vi "Evaluate Single Solution.vi"(7 "Processing Times (Rows Mach.Cols Jobs)":u16[][](array[numeric]), 9 "Schedule":u16[](array[numeric]), 10 "Number of Jobs":i32, 11 "Number of Machines":i32) -> (3 "Gannt Chart Out":T1[][](array[typedef]))   [LabVIEW 2013, in "GA.lvclass"]
uses:
  GA.lvclass
  Controls/GanntChart_Element.ctl
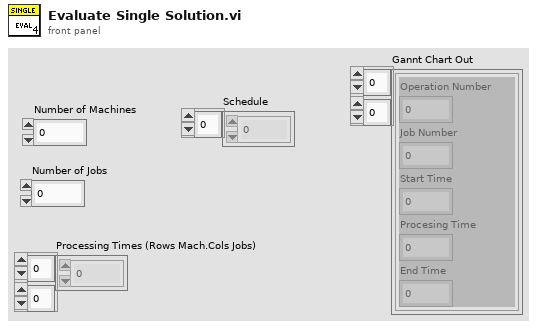
[diagram p1: front panel]
types:
  T1 = typedef "GanntChart_Element.ctl" = cluster{"Operation Number":i32, "Job Number":i32, "Start Time":i32, "Procesing Time":u16, "End Time":i32}
  T2 = typedef "Time_Interval_List_Element.ctl" = cluster{"Start Time":i32, "End Time":i32}
  T3 = typedef "Gap.ctl" = cluster{"Gap Start Time":i32, "Gap End Time":i32, "Gap Index":i32}
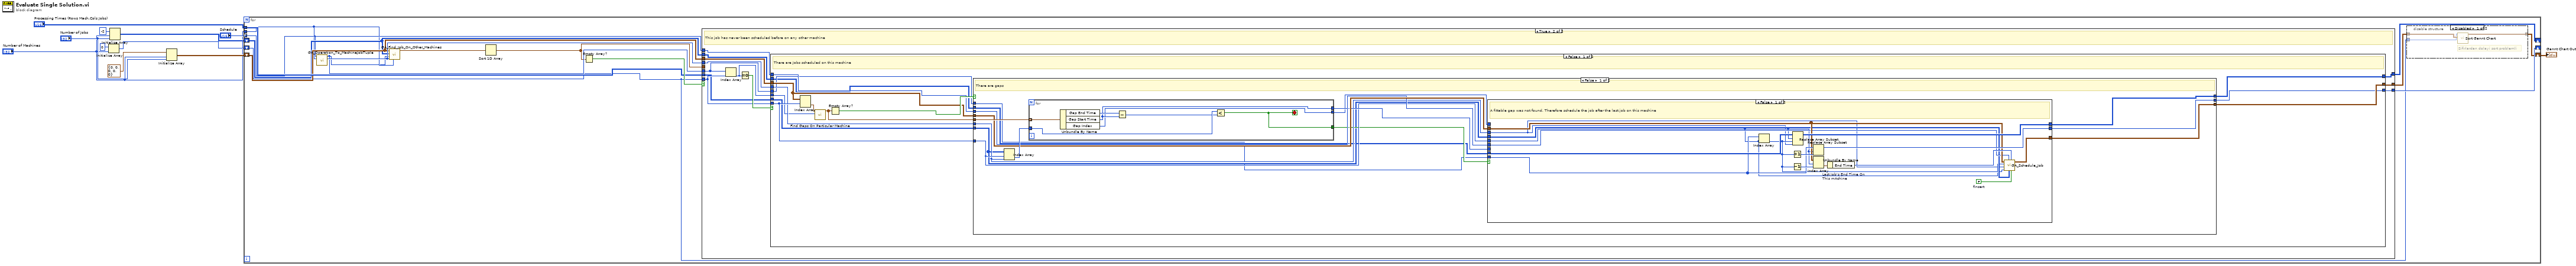
[diagram p0: block diagram]
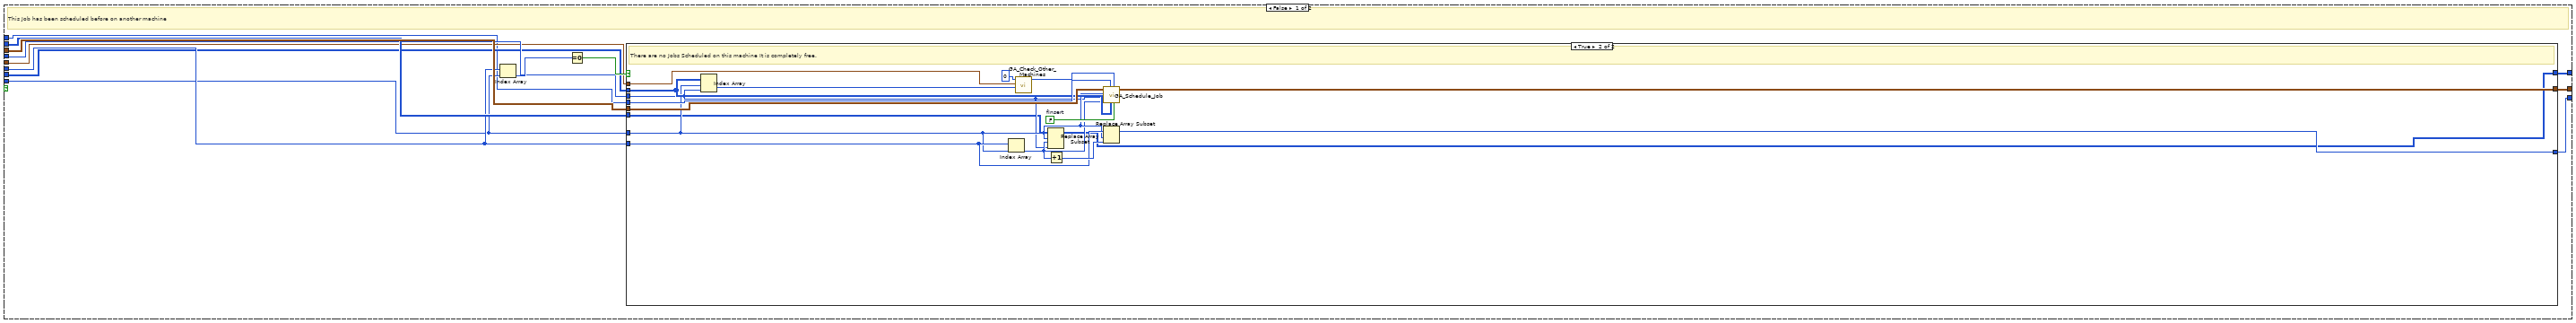
[diagram p3: hidden frame]
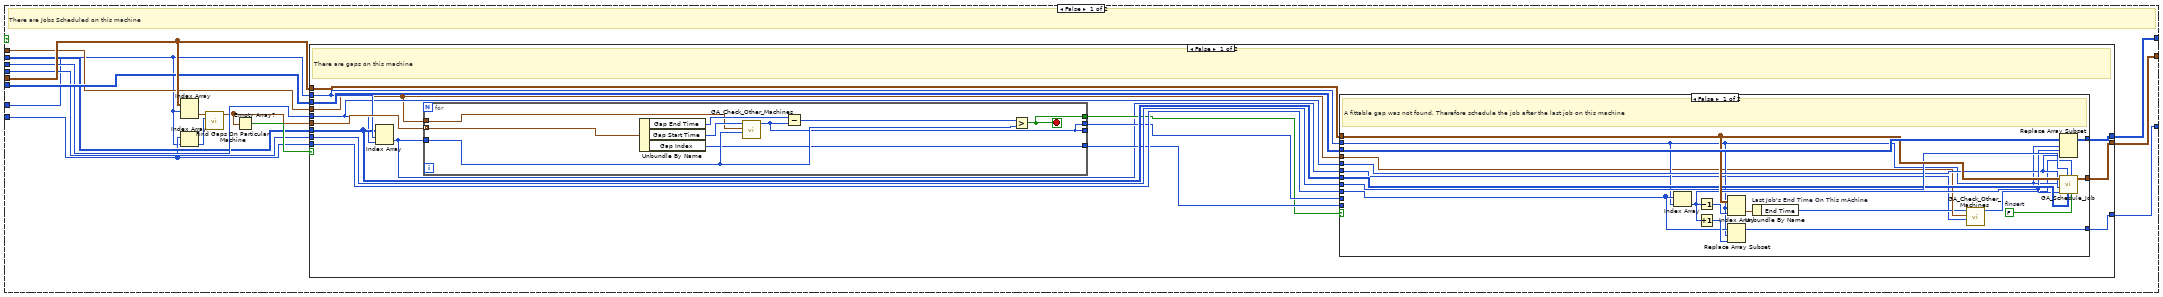
[diagram p4: hidden frame]
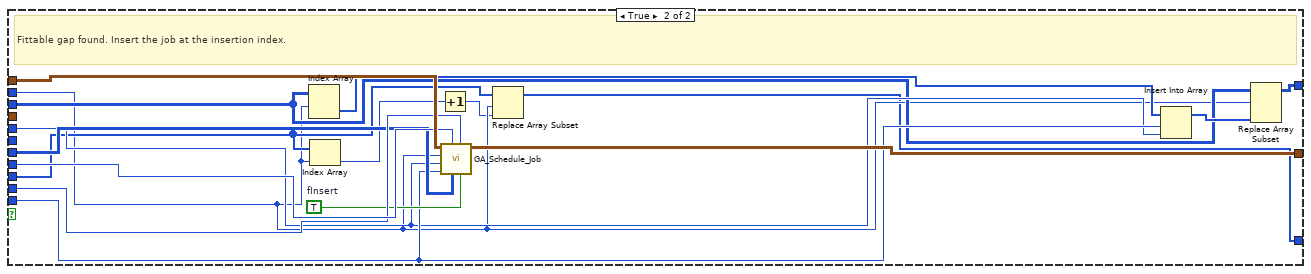
[diagram p5: hidden frame]
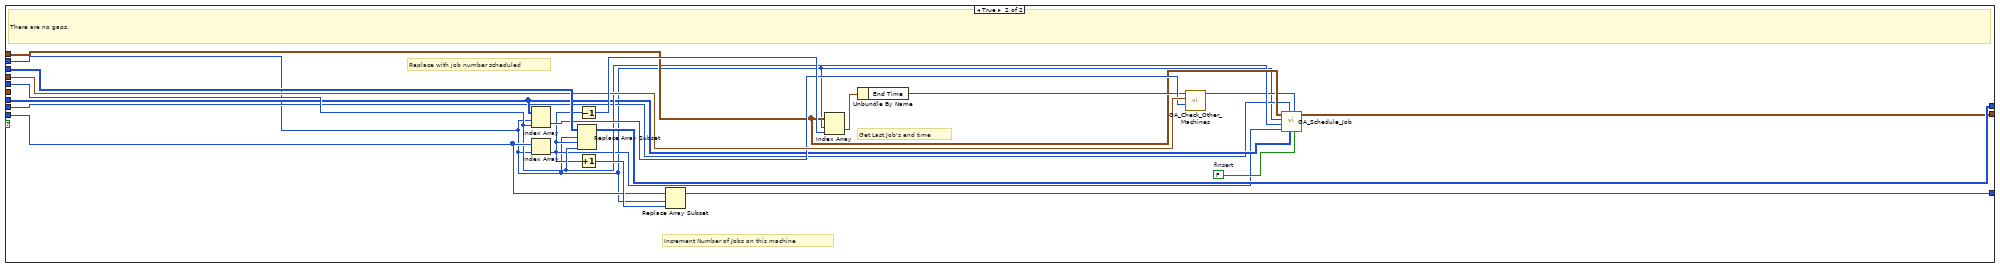
[diagram p6: hidden frame]
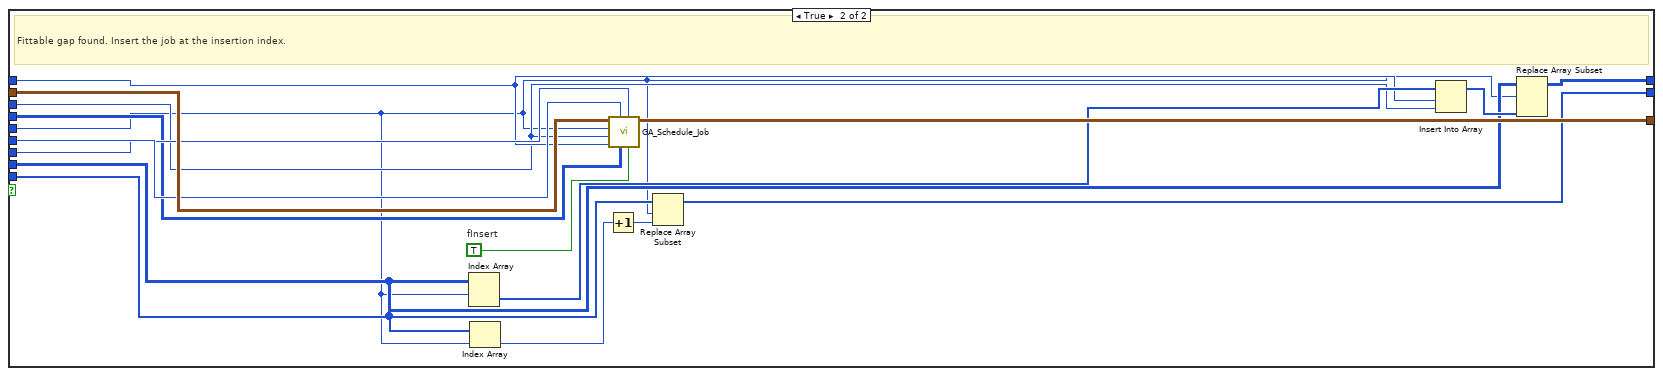
[diagram p7: hidden frame]
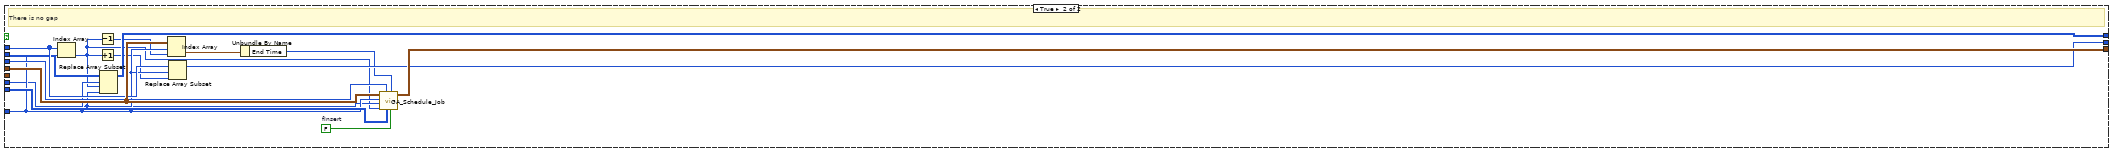
[diagram p8: hidden frame]
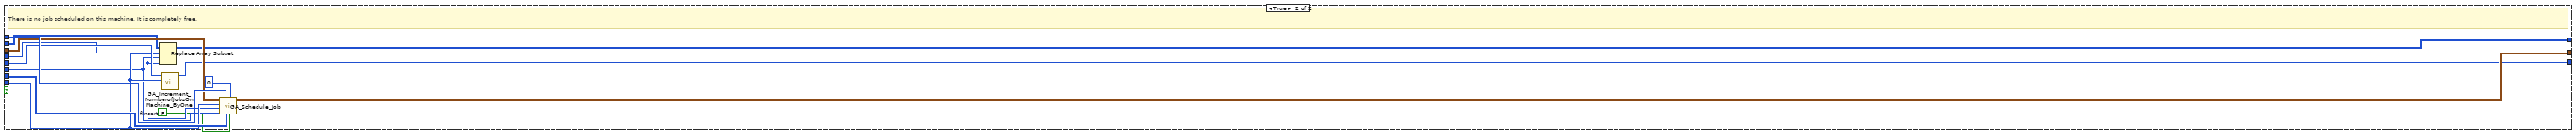
[diagram p9: hidden frame]
diagram:
  n1 = Initialize Array(0, "Number of Machines") -> (w2:i32[])
  n2 = Initialize Array(-2, "Number of Machines", "Number of Jobs") -> (w4:i32[][])
  n3 = Initialize Array(T1 {"Operation Number"=0, "Job Number"=0, "Start Time"=0, "Procesing Time"=0, "End Time"=0}, "Number of Machines", "Number of Jobs") -> (w7:T1[][])
  n4 = for {
    tunnel: "Schedule" -> [w19] mode=indexing
    tunnel: "Number of Machines" -> [w17]
    shift-right: [w12] -> w11
    shift-left: w7 -> [w23]
    tunnel: "Processing Times (Rows Mach.Cols Jobs)" -> [w25]
    shift-right: [w21] -> _
    shift-left: w4 -> [w22]
    shift-right: [w18] -> _
    shift-left: w2 -> [w20]
    n5 = call "GA_Operation_To_MachineJobTuple.vi"("Number of Machines"=w17, "Operation Number"=w19) -> ("Job No"=w24:i32, "Machine No"=w13:i32)  [unwired: 8 in]
    n6 = call "GA_Find_Job_On_Other_Machines.vi"("Number of Machines"=w17, "Job No"=w24, "Machine No"=w13, "Job Schedule on Machines"=w22, "Gannt Chart"=w23) -> ("Time Interval List"=w16:T2[])  [unwired: 6 in]
    n7 = Sort 1D Array(array=w16) -> (sorted array=w15:T2[])
    n8 = Empty Array?(array=w15) -> (empty?=w26:bool)
    n9 = case shown="True" w26 {
      tunnel: w25 -> [w32 w161]
      tunnel: w24 -> [w34 w162]
      tunnel: w23 -> [w42 w166]
      tunnel: [w41 w160] -> w14
      tunnel: w22 -> [w40 w157]
      tunnel: [w39 w156] -> w21
      tunnel: w13 -> [w35 w165]
      tunnel: w15 -> [w33 _]
      tunnel: w20 -> [w38 w159]
      tunnel: w19 -> [w31 w163]
      tunnel: [w37 w158] -> w18
      frame False {
        # "This Job has been scheduled before on another machine"
        n10 = Index Array(array=w38, index=w35) -> (element=w43:i32)
        n11 = Equal To 0?(x=w43) -> (x = 0?=w36:bool)
        n12 = case shown="True" w36 {
          tunnel: [w55 w151] -> w41
          tunnel: w42 -> [w56 w152]
          tunnel: w40 -> [w54 w140]
          tunnel: [w53 w139] -> w39
          tunnel: w38 -> [w47 w145]
          tunnel: [w52 w144] -> w37
          tunnel: w35 -> [w46 w143]
          tunnel: w34 -> [w51 w141]
          tunnel: w33 -> [w50 w155]
          tunnel: w32 -> [w49 w147]
          tunnel: w31 -> [w48 w149]
          frame False {
            # "There are Jobs Scheduled on this machine"
            n13 = Index Array(array=w56, index (row)=w46) -> (element=w58:T1[])  [unwired: 1 in]
            n14 = Index Array(array=w47, index=w46) -> (element=w45:i32)
            n15 = call "Find Gaps On Particular Machine.vi"("Number of Scheduled Jobs on This Machine"=w45, "Gannt Chart For Machine In"=w58) -> ("Gaps"=w44:T3[])  [unwired: 9 in]
            n16 = Empty Array?(array=w44) -> (empty?=w57:bool)
            n17 = case shown="False" w57 {
              tunnel: w56 -> [w69 w127]
              tunnel: [w68 w126] -> w55
              tunnel: [w70 w131] -> w53
              tunnel: w54 -> [w71 w132]
              tunnel: [w72 w133] -> w52
              tunnel: w47 -> [w73 w134]
              tunnel: w46 -> [w66 w120]
              tunnel: w51 -> [w64 w125]
              tunnel: w50 -> [w61 w130]
              tunnel: w49 -> [w65 w124]
              tunnel: w48 -> [w67 w123]
              tunnel: w44 -> [w74 _]
              frame False {
                # "There are gaps on this machine"
                n18 = Index Array(array=w65, index (row)=w66, index (col)=w64) -> (element=w59:u16)
                n19 = for {
                  tunnel: w74 -> [w114] mode=indexing
                  tunnel: w59 -> [w118]
                  tunnel: [w112] -> w63
                  tunnel: [w116] -> w62
                  tunnel: w61 -> [w115]
                  tunnel: [w112] -> _
                  tunnel: [w111] -> w60
                  stop <- w111 stop-if-true
                  n20 = Unbundle By Name(w114) -> ("Gap End Time"=w119:i32, "Gap Start Time"=w117:i32, "Gap Index"=w116:i32)
                  n21 = call "GA_Check_Other_Machines.vi"("Processing Time of the Job on This Machine"=w118, "Time Interval List"=w115, "Current Machine Available Time"=w117) -> ("Time to schedule"=w112:i32)  [unwired: 8 in]
                  n22 = Subtract(x=w119, y=w112) -> (x-y=w113:i32)
                  n23 = Greater?(x=w113, y=w118) -> (0:w111:bool)
                }
                n24 = case shown="False" w60 {
                  tunnel: w69 -> [w85 w110]
                  tunnel: [w84 w109] -> w68
                  tunnel: w67 -> [w83 w108]
                  tunnel: w63 -> [_ w107]
                  tunnel: w66 -> [w79 w96]
                  tunnel: w64 -> [w80 w102]
                  tunnel: w65 -> [w82 w106]
                  tunnel: w62 -> [_ w103]
                  tunnel: w71 -> [w91 w100]
                  tunnel: w73 -> [w87 w97]
                  tunnel: [w90 w99] -> w70
                  tunnel: [w86 w94] -> w72
                  tunnel: w61 -> [w78 _]
                  tunnel: w59 -> [w76 _]
                  frame False {
                    w92 = FALSE  # fInsert
                    # "A fittable gap was not found. Therefore schedule the job after the last job on this machine"
                    n25 = Index Array(array=w87, index=w79) -> (element=w81:i32)
                    n26 = Decrement(x=w81) -> (x-1=w89:i32)
                    n27 = Increment(x=w81) -> (x+1=w93:i32)
                    n28 = Index Array(array=w85, index (row)=w79, index (col)=w89) -> (element=w88:T1)
                    n29 = Replace Array Subset(array=w87, new element=w93, index=w79) -> (w86:i32[])
                    n30 = Unbundle By Name "Last Job's End Time On This mAchine"(w88) -> ("End Time"=w77:i32)
                    n31 = call "GA_Check_Other_Machines.vi"("Processing Time of the Job on This Machine"=w76, "Time Interval List"=w78, "Current Machine Available Time"=w77) -> ("Time to schedule"=w75:i32)  [unwired: 8 in]
                    n32 = Replace Array Subset(array=w91, new element=w80, index (row)=w79, index (col)=w81) -> (w90:i32[][])
                    n33 = call "GA_Schedule_Job.vi"("fInsert"=w92, "Start Time"=w75, "Processing Times"=w82, "Operation"=w83, "Index to schedule/Insert"=w81, "Job Number"=w80, "Machine No"=w79, "Gannt Chart In"=w85) -> ("Gannt Chart Out"=w84:T1[][])  [unwired: 3 in]
                  }
                  frame True {
                    w105 = TRUE  # fInsert
                    # "Fittable gap found. Insert the job at the insertion index."
                    n34 = Index Array(array=w100, index (row)=w96) -> (element=w104:i32[])  [unwired: 1 in]
                    n35 = Index Array(array=w97, index=w96) -> (element=w98:i32)
                    n36 = Increment(x=w98) -> (x+1=w95:i32)
                    n37 = call "GA_Schedule_Job.vi"("fInsert"=w105, "Start Time"=w107, "Processing Times"=w106, "Operation"=w108, "Index to schedule/Insert"=w103, "Job Number"=w102, "Machine No"=w96, "Gannt Chart In"=w110) -> ("Gannt Chart Out"=w109:T1[][])  [unwired: 3 in]
                    n38 = Replace Array Subset(array=w97, new element=w95, index=w96) -> (w94:i32[])
                    n39 = Insert Into Array(array=w104, index=w103, new element=w102) -> (w101:i32[])
                    n40 = Replace Array Subset(array=w100, new element=w101, index (row)=w96) -> (w99:i32[][])  [unwired: 1 in]
                  }
                }
              }
              frame True {
                w136 = FALSE  # fInsert
                # "Get Last Job's end time"
                # "Increment Number of Jobs on this machine"
                # "Replace with job number scheduled"
                # "There are no gaps."
                n41 = Index Array(array=w124, index (row)=w120, index (col)=w125) -> (element=w129:u16)
                n42 = Index Array(array=w134, index=w120) -> (element=w121:i32)
                n43 = Replace Array Subset(array=w132, new element=w125, index (row)=w120, index (col)=w121) -> (w131:i32[][])
                n44 = Decrement(x=w121) -> (x-1=w138:i32)
                n45 = Increment(x=w121) -> (x+1=w137:i32)
                n46 = Replace Array Subset(array=w134, new element=w137, index=w120) -> (w133:i32[])
                n47 = Index Array(array=w127, index (row)=w120, index (col)=w138) -> (element=w135:T1)
                n48 = Unbundle By Name(w135) -> ("End Time"=w128:i32)
                n49 = call "GA_Check_Other_Machines.vi"("Processing Time of the Job on This Machine"=w129, "Time Interval List"=w130, "Current Machine Available Time"=w128) -> ("Time to schedule"=w122:i32)  [unwired: 8 in]
                n50 = call "GA_Schedule_Job.vi"("fInsert"=w136, "Start Time"=w122, "Processing Times"=w124, "Operation"=w123, "Index to schedule/Insert"=w121, "Job Number"=w125, "Machine No"=w120, "Gannt Chart In"=w127) -> ("Gannt Chart Out"=w126:T1[][])  [unwired: 3 in]
              }
            }
          }
          frame True {
            w150 = FALSE  # fInsert
            # "There are no Jobs Scheduled on this machine It is completely free."
            n51 = Index Array(array=w147, index (row)=w143, index (col)=w141) -> (element=w153:u16)
            n52 = Index Array(array=w145, index=w143) -> (element=w142:i32)
            n53 = call "GA_Check_Other_Machines.vi"("Processing Time of the Job on This Machine"=w153, "Time Interval List"=w155, "Current Machine Available Time"=0) -> ("Time to schedule"=w148:i32)  [unwired: 8 in]
            n54 = Replace Array Subset(array=w140, new element=w141, index (row)=w143, index (col)=w142) -> (w139:i32[][])
            n55 = Increment(x=w142) -> (x+1=w146:i32)
            n56 = call "GA_Schedule_Job.vi"("fInsert"=w150, "Start Time"=w148, "Processing Times"=w147, "Operation"=w149, "Index to schedule/Insert"=w142, "Job Number"=w141, "Machine No"=w143, "Gannt Chart In"=w152) -> ("Gannt Chart Out"=w151:T1[][])  [unwired: 3 in]
            n57 = Replace Array Subset(array=w145, new element=w146, index=w143) -> (w144:i32[])
          }
        }
      }
      frame True {
        # "This job has never been scheduled before on any other machine"
        n58 = Index Array(array=w159, index=w165) -> (element=w164:i32)
        n59 = Equal To 0?(x=w164) -> (x = 0?=w167:bool)
        n60 = case shown="False" w167 {
          tunnel: w166 -> [w178 w262]
          tunnel: w165 -> [w179 w258]
          tunnel: w164 -> [w168 w257]
          tunnel: w163 -> [w176 w263]
          tunnel: w162 -> [w175 w256]
          tunnel: w161 -> [w174 w265]
          tunnel: [w177 w264] -> w160
          tunnel: [w171 w260] -> w158
          tunnel: w159 -> [w172 w261]
          tunnel: w157 -> [w170 w259]
          tunnel: [w169 w255] -> w156
          frame False {
            # "There are Jobs scheduled on this machine"
            n61 = Index Array(array=w178, index (row)=w179) -> (element=w181:T1[])  [unwired: 1 in]
            n62 = call "Find Gaps On Particular Machine.vi"("Number of Scheduled Jobs on This Machine"=w168, "Gannt Chart For Machine In"=w181) -> ("Gaps"=w173:T3[])  [unwired: 9 in]
            n63 = Empty Array?(array=w173) -> (empty?=w180:bool)
            n64 = case shown="False" w180 {
              tunnel: w178 -> [w194 w250]
              tunnel: w172 -> [w183 w248]
              tunnel: w179 -> [w190 w245]
              tunnel: [w193 w252] -> w177
              tunnel: w176 -> [w192 w251]
              tunnel: w175 -> [w189 w244]
              tunnel: w174 -> [w187 w249]
              tunnel: w173 -> [w196 _]
              tunnel: [w182 w247] -> w171
              tunnel: w170 -> [w185 w246]
              tunnel: [w184 w243] -> w169
              frame False {
                # "There are gaps"
                n65 = Index Array(array=w187, index (row)=w190, index (col)=w189) -> (element=w195:u16)
                n66 = for {
                  tunnel: w196 -> [w236] mode=indexing
                  tunnel: w195 -> [w234]
                  tunnel: [w232] -> w191
                  tunnel: [w231] -> w188
                  tunnel: [w230] -> w186
                  stop <- w231 stop-if-true
                  n67 = Unbundle By Name(w236) -> ("Gap End Time"=w235:i32, "Gap Start Time"=w232:i32, "Gap Index"=w230:i32)
                  n68 = Subtract(x=w235, y=w232) -> (x-y=w233:i32)
                  n69 = Less?(x=w234, y=w233) -> (x < y?=w231:bool)
                }
                n70 = case shown="False" w188 {
                  tunnel: w194 -> [w203 w229]
                  tunnel: [w202 w228] -> w193
                  tunnel: w192 -> [w201 w227]
                  tunnel: w191 -> [_ w226]
                  tunnel: w190 -> [w198 w215]
                  tunnel: w189 -> [w197 w221]
                  tunnel: w187 -> [w200 w225]
                  tunnel: w186 -> [_ w222]
                  tunnel: w185 -> [w210 w219]
                  tunnel: w183 -> [w206 w216]
                  tunnel: [w209 w218] -> w184
                  tunnel: [w205 w213] -> w182
                  frame False {
                    w211 = FALSE  # fInsert
                    # "A fittable gap was not found. Therefore schedule the job after the last job on this machine"
                    n71 = Index Array(array=w206, index=w198) -> (element=w199:i32)
                    n72 = Increment(x=w199) -> (x+1=w212:i32)
                    n73 = Decrement(x=w199) -> (x-1=w208:i32)
                    n74 = Replace Array Subset(array=w210, new element=w197, index (row)=w198, index (col)=w199) -> (w209:i32[][])
                    n75 = Replace Array Subset(array=w206, new element=w212, index=w198) -> (w205:i32[])
                    n76 = Index Array(array=w203, index (row)=w198, index (col)=w208) -> (element=w207:T1)
                    n77 = Unbundle By Name "Last Job's End Time On This mAchine"(w207) -> ("End Time"=w204:i32)
                    n78 = call "GA_Schedule_Job.vi"("fInsert"=w211, "Start Time"=w204, "Processing Times"=w200, "Operation"=w201, "Index to schedule/Insert"=w199, "Job Number"=w197, "Machine No"=w198, "Gannt Chart In"=w203) -> ("Gannt Chart Out"=w202:T1[][])  [unwired: 3 in]
                  }
                  frame True {
                    w224 = TRUE  # fInsert
                    # "Fittable gap found. Insert the job at the insertion index."
                    n79 = Index Array(array=w219, index (row)=w215) -> (element=w223:i32[])  [unwired: 1 in]
                    n80 = Index Array(array=w216, index=w215) -> (element=w217:i32)
                    n81 = Increment(x=w217) -> (x+1=w214:i32)
                    n82 = call "GA_Schedule_Job.vi"("fInsert"=w224, "Start Time"=w226, "Processing Times"=w225, "Operation"=w227, "Index to schedule/Insert"=w222, "Job Number"=w221, "Machine No"=w215, "Gannt Chart In"=w229) -> ("Gannt Chart Out"=w228:T1[][])  [unwired: 3 in]
                    n83 = Replace Array Subset(array=w216, new element=w214, index=w215) -> (w213:i32[])
                    n84 = Insert Into Array(array=w223, index=w222, new element=w221) -> (w220:i32[])
                    n85 = Replace Array Subset(array=w219, new element=w220, index (row)=w215) -> (w218:i32[][])  [unwired: 1 in]
                  }
                }
              }
              frame True {
                w237 = FALSE  # fInsert
                # "There is no gap"
                n86 = Index Array(array=w248, index=w245) -> (element=w238:i32)
                n87 = Decrement(x=w238) -> (x-1=w242:i32)
                n88 = Increment(x=w238) -> (x+1=w239:i32)
                n89 = Replace Array Subset(array=w246, new element=w244, index (row)=w245, index (col)=w238) -> (w243:i32[][])
                n90 = Index Array(array=w250, index (row)=w245, index (col)=w242) -> (element=w241:T1)
                n91 = Replace Array Subset(array=w248, new element=w239, index=w245) -> (w247:i32[])
                n92 = Unbundle By Name(w241) -> ("End Time"=w240:i32)
                n93 = call "GA_Schedule_Job.vi"("fInsert"=w237, "Start Time"=w240, "Processing Times"=w249, "Operation"=w251, "Index to schedule/Insert"=w238, "Job Number"=w244, "Machine No"=w245, "Gannt Chart In"=w250) -> ("Gannt Chart Out"=w252:T1[][])  [unwired: 3 in]
              }
            }
          }
          frame True {
            w253 = FALSE  # fInsert
            # "There is no job scheduled on this machine. It is completely free."
            n94 = Replace Array Subset(array=w259, new element=w256, index (row)=w258, index (col)=w257) -> (w255:i32[][])
            n95 = call "GA_Increment_NumberofJobsOn Machine_ByOne.vi"("Machine Number"=w258, "Number of Jobs Scheduled On Machines in"=w261) -> ("Number of Jobs Scheduled On Machines out"=w260:i32[])  [unwired: 9 in]
            n96 = call "GA_Schedule_Job.vi"("fInsert"=w253, "Start Time"=0, "Processing Times"=w265, "Operation"=w263, "Index to schedule/Insert"=w257, "Job Number"=w256, "Machine No"=w258, "Gannt Chart In"=w262) -> ("Gannt Chart Out"=w264:T1[][])  [unwired: 3 in]
          }
        }
      }
    }
    n97 = disable-structure shown="Disabled" {
      disable-tunnel: w14 -> [w29 w30]
      disable-tunnel: w13 -> [w28 _]
      disable-tunnel: [w27 w30] -> w12
      frame Disabled {
        # "Sifirlardan dolayi sort problemli"
        n98 = call "Sort Gannt Chart.vi"("Gannt Chart  in"=w29, "Machine Number"=w28) -> ("Gannt Chart Out out"=w27:T1[][])  [unwired: 9 in]
      }
      frame Enabled {
      }
    }
  }
  "Gannt Chart Out" <- w11
